vi "Bytes to U16s1.vi"(11 "bytes":u8[](array[numeric])) -> (3 "registers":u16[](array[numeric]))   [LabVIEW 2021, in "NI_modbus_upd.lvlib"]
uses:
  NI_modbus_upd.lvlib
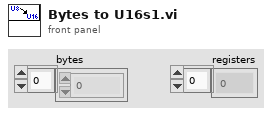
[diagram p1: front panel]
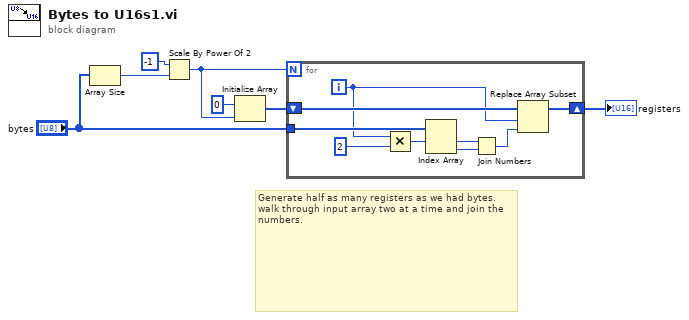
[diagram p0: block diagram]
diagram:
  # "Generate half as many registers as we had bytes. walk through input array two at a time and join the numbers."
  n1 = Array Size(array="bytes") -> (size(s)=w6:i32)
  n2 = Scale By Power Of 2(n=i16 -1, x=w6) -> (x*2^n=w4:i32)
  n3 = Initialize Array(u16 0 ("Numeric"), w4) -> (w2:u16[])
  n4 = for {
    N: w4 -> [_]
    tunnel: "bytes" -> [w14]
    shift-right: [w16] -> w1
    shift-left: w2 -> [w15]
    i -> [w8]
    n5 = Multiply(x=w8, y=2 ("x")) -> (x*y=w12:i32)
    n6 = Index Array(array=w14, index #1=w12) -> (element #1=w11:u8, element #2=w10:u8)  [unwired: 1 in]
    n7 = Join Numbers(hi=w11, lo=w10) -> ((hi.lo)=w9:u16)
    n8 = Replace Array Subset(array=w15, new element=w9, index=w8) -> (w16:u16[])
  }
  "registers" <- w1
